vi "SRV_Get TCP Connection.vi"(8 "error in (no error)":errorcluster, 11 "IP address":string) -> (0 "error out":errorcluster, 3 "connection ID":refnum<k5>)   [LabVIEW 2009]
doc: "Get a TCP Connection."
uses:
  SubVIs/SRVGlobals.vi
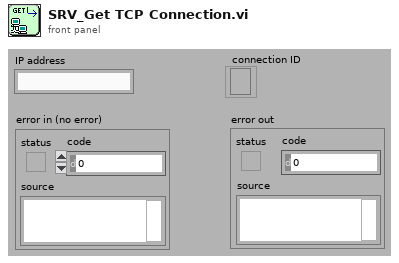
[diagram p1: front panel]
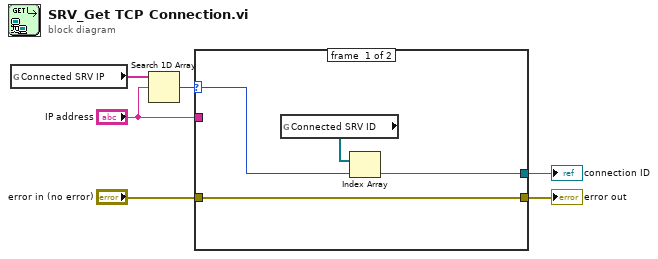
[diagram p0: block diagram]
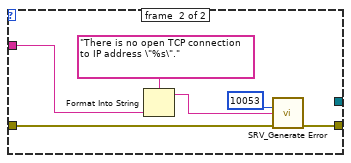
[diagram p2: hidden frame]
diagram:
  n1 = global read "SRVGlobals.vi" "Connected SRV IP"() -> (w2:string[])
  n2 = Search 1D Array(1D array=w2, element="IP address") -> (index of element=w4:i32)  [unwired: 1 in]
  n3 = case shown="Default" w4 {
    selector: w4 -> [w10 _]
    tunnel: [w8 _] -> w6
    tunnel: [w7 w16] -> w5
    tunnel: "error in (no error)" -> [w7 w15]
    tunnel: "IP address" -> [_ w13]
    frame #0 {
      n4 = global read "SRVGlobals.vi" "Connected SRV ID"() -> (w9:refnum<k5>[])
      n5 = Index Array(array=w9, index=w10) -> (element=w8:refnum<k5>)
    }
    frame #1 {
      n6 = Format Into String(format string="There is no open TCP connection to IP address \"%s\".", w13) -> (resulting string=w12:string)  [unwired: 2 in, 1 out]
      n7 = call "SRV_Generate Error.vi"("code (42: generic error)"=10053, "Message"=w12, "error in (no error)"=w15) -> ("error out"=w16:errorcluster)  [unwired: 12 in]
    }
  }
  "error out" <- w5
  "connection ID" <- w6
